vi "trial code.vi"() -> ()   [LabVIEW 2025]
uses:
  <vilib>/Instr/_visa.llb/VISA Configure Serial Port (Instr).vi
  <vilib>/addons/control/pid/NI_PID_pid.lvlib
  <vilib>/addons/control/pid/pid.llb/PID (DBL).vi
  <vilib>/numeric/Random Number (Range) DBL.vi
panel:
  in  "lower bound (0)":dbl
  in  "Stroke 2":dbl
  out "error out":errorcluster
  out "Stroke RAW":dbl
  out "Stroke Tare":dbl
  in  "Boolean":bool
  in  "PID SEND":bool
  in  "PID ON":bool
  in  "Stop 3":bool
  out "output Vpp":dbl
  in  "input variable":dbl=1.0
  in  "Stop 2":bool
  out "Stroke":dbl
  out "cof":dbl
  out "Friction":dbl
  out "pizo raw":dbl
  out "LVDT Peak":dbl
  out "LVDT MAX":dbl
  out "LVDT MIN":dbl
  in  "Stroke PID Gains 2":T1={"Proportional Gain (Kc)"=200.0, "Integral Time (Ti, min)"=0.02, "Derivative Time (Td, min)"=0.0}
  in  "STROKE GAIN :":dbl=700.0 caption="Stroke Gain :"
  in  "Set Strk":dbl=1.0 caption="STROKE LENGTH" min=1.0 max=1.0 step=1.0 format="%.3f"
  in  "PID Rst":bool=TRUE
  out "Stroke PID OUT":dbl(slide)=-13.483146067415703 scale=-600.0..600.0
  out "stop cmd":bool
  out "st gain":string="0000"
  out "PID Out":u8(slide) scale=0.0..4095.0
  out "start en":bool=TRUE
  in  "command":string
  in  "Stop":bool
  in  "Com Port 2":refnum<visa-resource-name>="COM9" caption="C2 :"
  out "Residual Uno 2":string
  out "Port 1 Error 2":errorcluster={"status"=TRUE, "code"=-1073807343, "source"="Property Node (arg 1) in VISA Configure Serial Port (Instr).vi->Winducom 2010--std ed hfrr-wo1768-V18.vi"}
  out "Uno Stroke":string
  out "Sps 4":dbl
  out "Port 1a 2":bool caption="Port 1 a"
  out "Port 2":u32(graph)
  out "Error Uno 2":errorcluster={"status"=TRUE, "code"=-1073807343, "source"="Property Node (arg 1) in VISA Configure Serial Port (Instr).vi->Winducom 2010--std ed hfrr-wo1768-V18.vi"}
  out "Port 4":bool=TRUE caption="Port 1"
  in  "Re-initialize Port1 2":bool
  out "Residual Uno":string
  out "Port 1 Error":errorcluster={"status"=TRUE, "code"=-1073807343, "source"="Property Node (arg 1) in VISA Configure Serial Port (Instr).vi->Winducom 2010--std ed hfrr-wo1768-V18.vi"}
  out "due":string
  out "Sps 3":dbl
  out "Port 1a":bool caption="Port 1 a"
  out "Port 1":u32(graph)
  out "Error Uno":errorcluster={"status"=TRUE, "code"=-1073807343, "source"="Property Node (arg 1) in VISA Configure Serial Port (Instr).vi->Winducom 2010--std ed hfrr-wo1768-V18.vi"}
  out "Port 3":bool=TRUE caption="Port 1"
  in  "Re-initialize Port1":bool
  out "FF buffer":dbl[](graph)
  in  "Com Port 1":refnum<visa-resource-name>="COM7" caption="C1 :"
  out "Test \nStatus":bool caption="Test Status"
types:
  T1 = cluster{"Proportional Gain (Kc)":dbl, "Integral Time (Ti, min)":dbl, "Derivative Time (Td, min)":dbl}
  T2 = cluster{"Read Heave and Surge":string, "Bytes at Heave Port":dbl, "Heave and Surge COM Port:":refnum<visa-resource-name>, "Com Port 2":refnum<visa-resource-name>, "Residual Due":string, "Heave COM Status 2":bool, "Heave COM Status":bool, "Port 2":bool, "Sway PPR":dbl, "Surge PPR":dbl, "Heave PPR":dbl, "Sway Pitch":dbl, "Surge Pitch":dbl, "Heave Pitch":dbl, "Sway Pulses/mm":dbl, "Surge Pulses/mm":dbl, "Heave Pulses/mm":dbl, "inner loop":dbl, "Read Heave and Surge 2":string, "String 36":string, "Write S":bool, "WriteCC1":string[], "Heave COM Loop":i32, "LastCom":string, "EXIT":bool, "Error Heave":errorcluster}
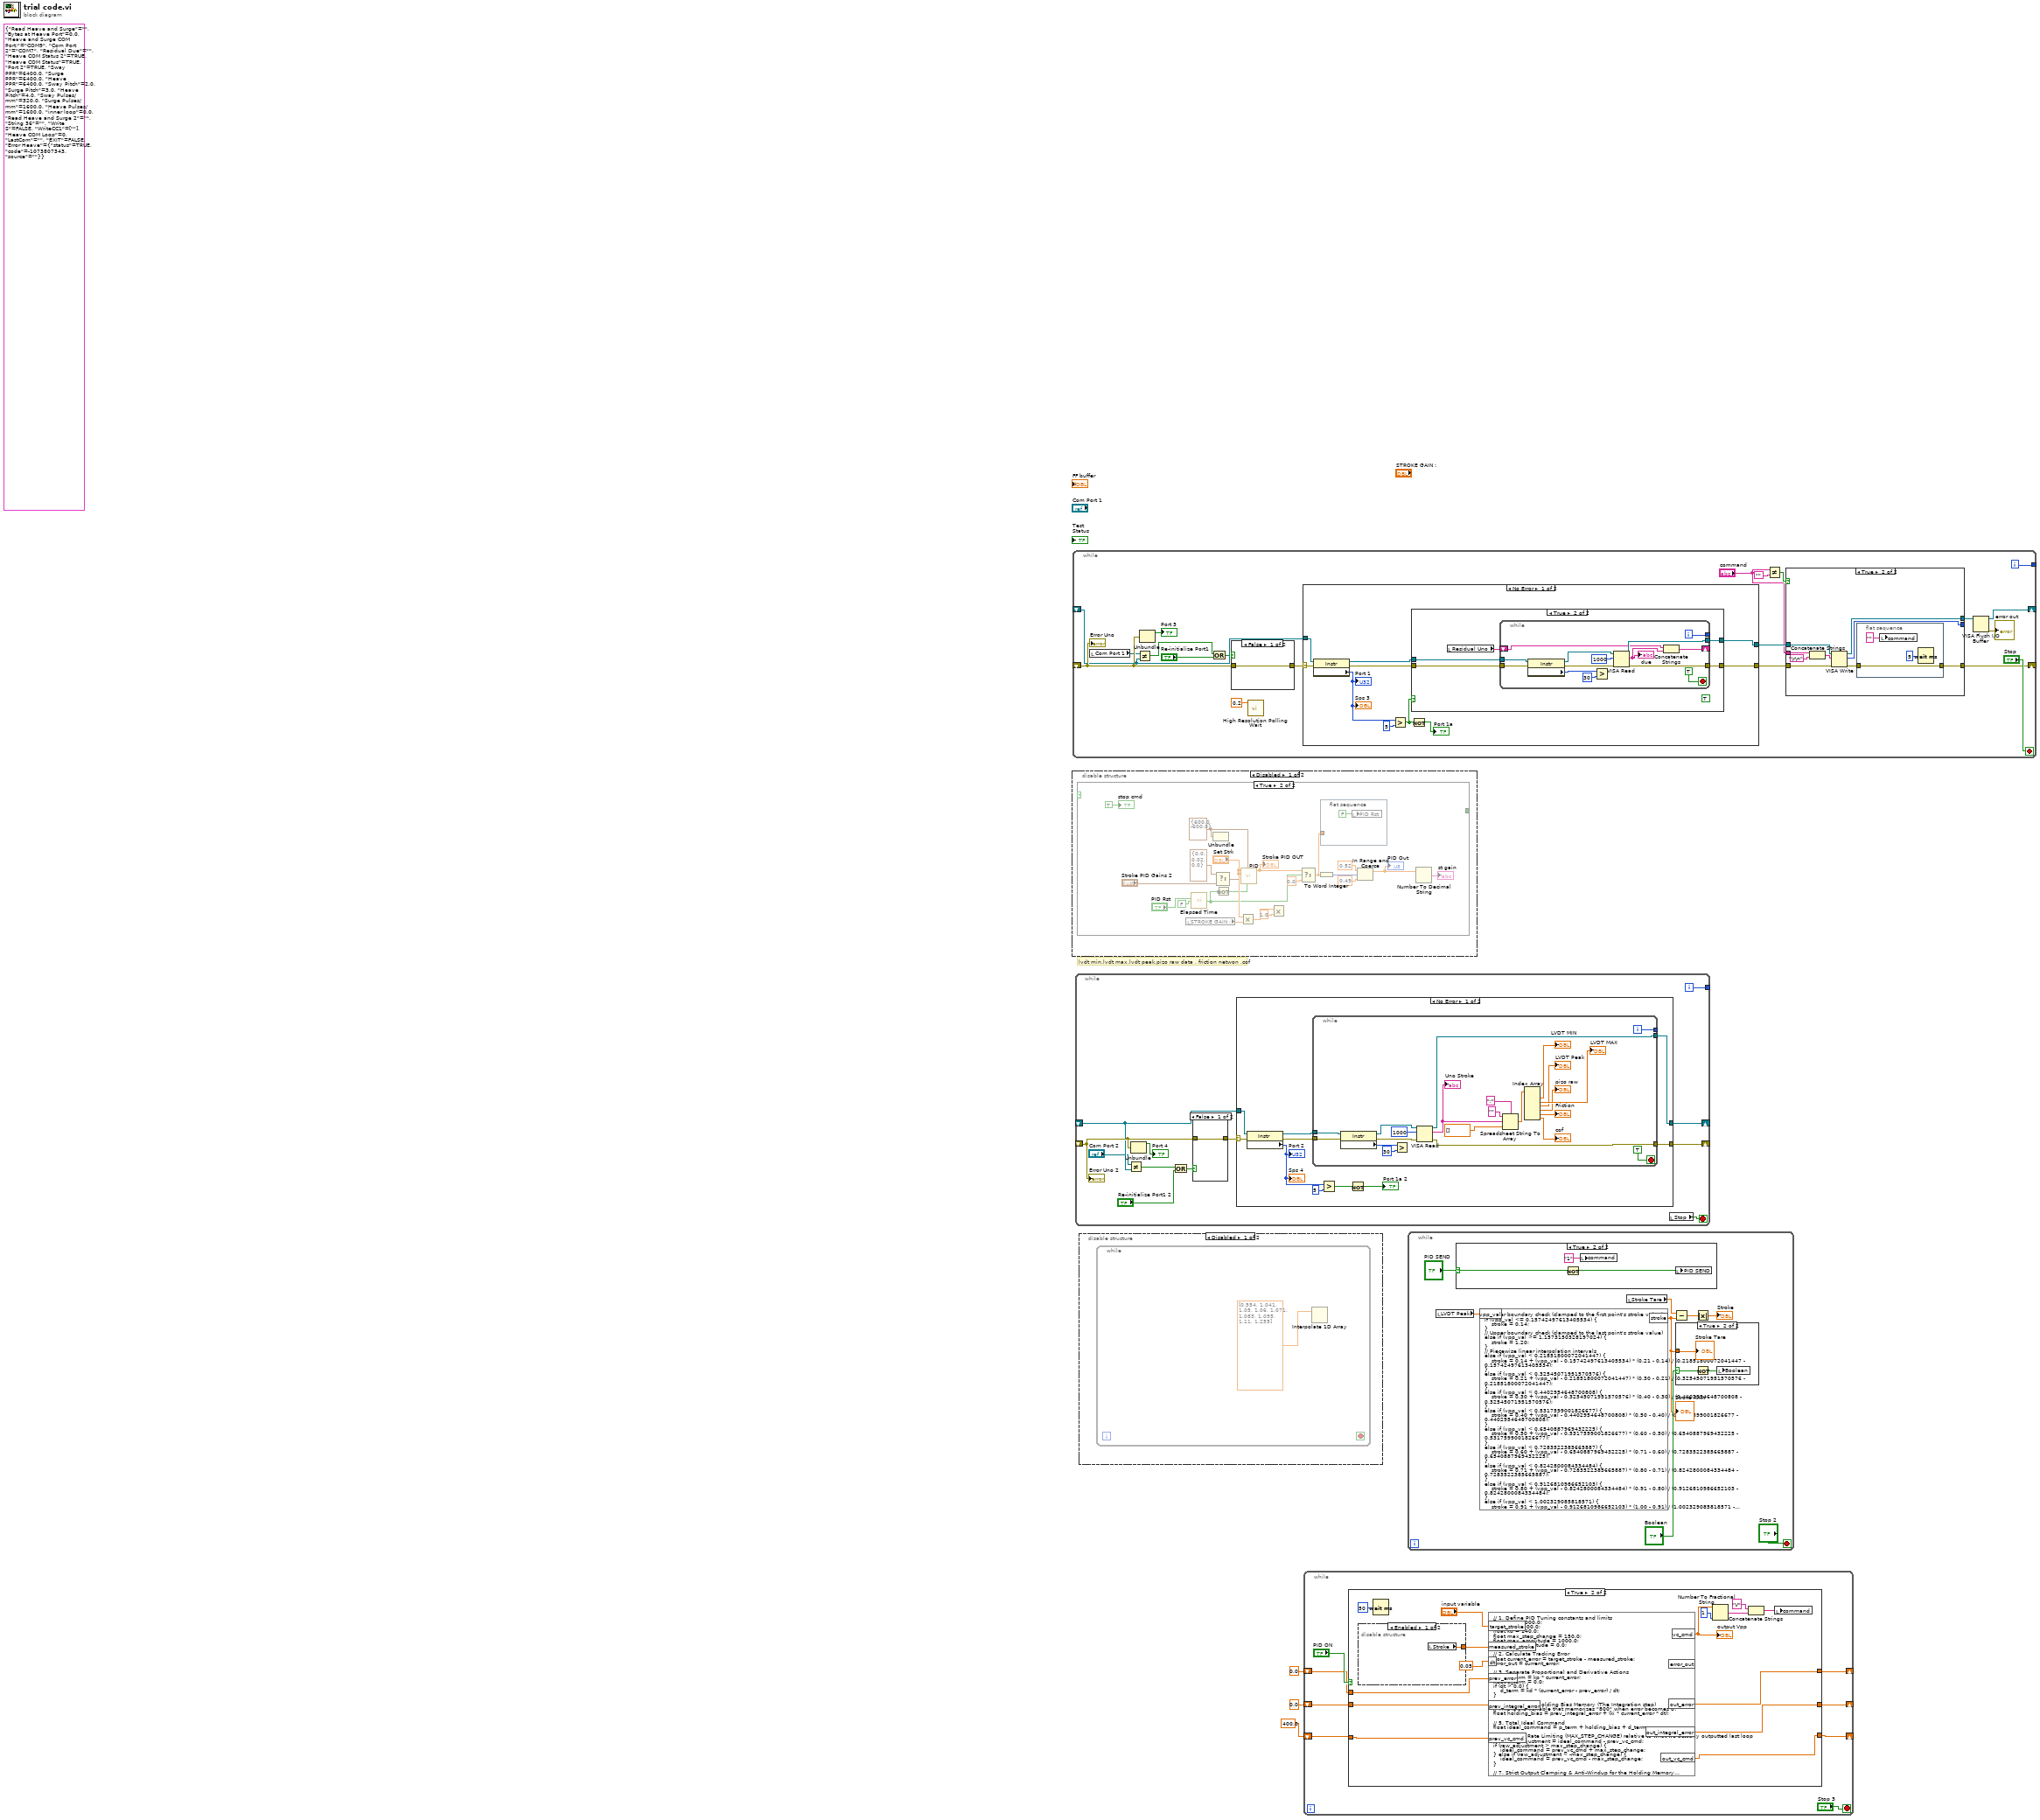
[diagram p0: block diagram]
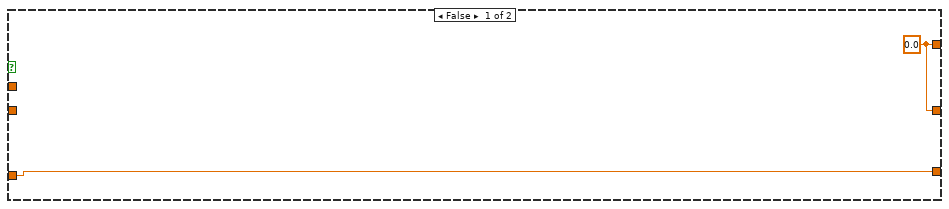
[diagram p2: hidden frame]
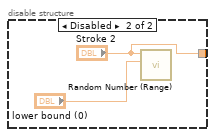
[diagram p3: hidden frame]
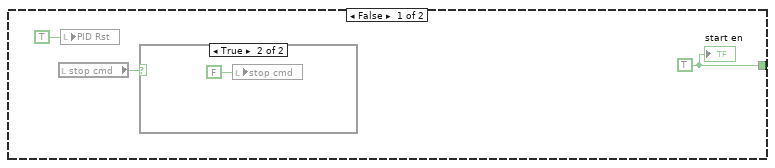
[diagram p7: hidden frame]
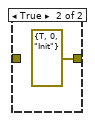
[diagram p10: hidden frame]
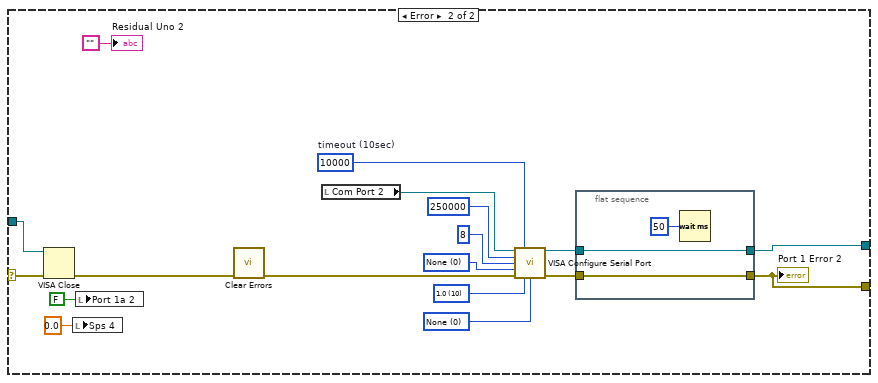
[diagram p11: hidden frame]
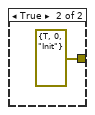
[diagram p13: hidden frame]
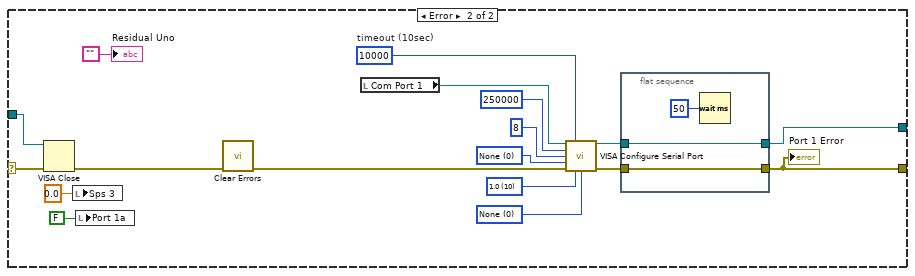
[diagram p15: hidden frame]
diagram:
  (unwired) T2 {"Read Heave and Surge"="", "Bytes at Heave Port"=0.0, "Heave and Surge COM Port:"="COM9", "Com Port 2"="COM7", "Residual Due"="", "Heave COM Status 2"=TRUE, "Heave COM Status"=TRUE, "Port 2"=TRUE, "Sway PPR"=6400.0, "Surge PPR"=6400.0, "Heave PPR"=6400.0, "Sway Pitch"=2.0, "Surge Pitch"=3.0, "Heave Pitch"=4.0, "Sway Pulses/mm"=320.0, "Surge Pulses/mm"=1600.0, "Heave Pulses/mm"=1600.0, "inner loop"=0.0, "Read Heave and Surge 2"="", "String 36"="", "Write S"=FALSE, "WriteCC1"=[""], "Heave COM Loop"=0, "LastCom"="", "EXIT"=FALSE, "Error Heave"={"status"=TRUE, "code"=-1073807343, "source"=""}}
  # "lvdt min,lvdt max,lvdt peak,pizo raw data , friction netwon ,cof"
  n1 = disable-structure shown="Disabled" {
    frame Disabled {
      n2 = case shown="True" {
        selector: _ -> [_ _]
        tunnel: [w4 _] -> _
        frame False {
          w4 = TRUE ("PID Rst")
          n3 = local read "stop cmd"() -> (w5:bool)
          n4 = local write "PID Rst"(TRUE ("PID Rst")) -> ()
          n5 = case shown="True" w5 {
            frame False {
            }
            frame True {
              n6 = local write "stop cmd"(FALSE ("stop cmd")) -> ()
            }
          }
          "start en" <- w4
        }
        frame True {
          w24 = cluster{"output high":dbl, "output low":dbl} {"output high"=600.0, "output low"=-600.0} ("output range")
          n7 = local read "STROKE GAIN :"() -> (w14:dbl)
          n8 = call "Elapsed Time"("Reset"="PID Rst", "Auto Reset"=FALSE) -> ("Time has Elapsed"=w21:bool)  [unwired: 10 in, 7 out]
          n9 = Unbundle(w24) -> ()  [unwired: 2 out]
          n10 = Select(t=T1 {"Proportional Gain (Kc)"=0.0, "Integral Time (Ti, min)"=0.02, "Derivative Time (Td, min)"=0.0} ("Stroke PID Gains"), f="Stroke PID Gains 2") -> (s? t:f=w11:T1)  [unwired: 1 in]
          n11 = Not(x=w21) -> (.not. x?=w20:bool)
          n12 = Multiply(x="Set Strk", y=w14) -> (x*y=w9:dbl)
          n13 = call-poly <vilib>:"PID.vi"("reinitialize? (F)"=w20, "output range"=w24, "PID gains"=w11, "process variable"="Set Strk", "setpoint"="Set Strk") -> ("output"=w19:dbl)  [unwired: 5 in, 1 out]
          "Stroke PID OUT" <- w19
          n14 = Multiply(x=w9, y=1.0) -> ()  [unwired: 1 out]
          n15 = Select(t=w19, s=w21, f=0.0) -> (s? t:f=w22:dbl)
          n16 = To Word Integer(number=w22) -> (16bit integer=w16:i16)
          n17 = flat-sequence {
            tunnel: w22 -> [_]
            frame #0 {
              n18 = local write "PID Rst"(FALSE ("PID Rst")) -> ()
            }
          }
          n19 = In Range and Coerce(upper limit=0.52 ("f"), x=w16, lower limit=0.49 ("f")) -> (coerced(x)=w13:dbl)  [unwired: 1 out]
          "PID Out" <- w13
          n20 = Number To Decimal String(number=w13) -> (decimal integer string=→"st gain":string)  [unwired: 1 in]
          "stop cmd" <- TRUE ("Auto Reset")
        }
      }
    }
    frame Enabled {
    }
  }
  n21 = while {
    shift-right: [w31] -> _
    shift-left: _ -> [w45]
    shift-right: [w36] -> _
    shift-left: _ -> [w47]
    tunnel: [w49] -> _
    i -> [w49]
    stop <- "Stop" stop-if-true
    n22 = local read "Com Port 1"() -> (w46:refnum<visa-resource-name>)
    n23 = Not Equal?(x=w46, y=w45) -> (x != y?=w44:bool)
    n24 = Unbundle(w47) -> ("status"=→"Port 3":bool)  [unwired: 2 out]
    n25 = Or(x=w44, y="Re-initialize Port1") -> (x .or. y?=w42:bool)
    n26 = case shown="False" w42 {
      tunnel: [w64 errorcluster {"status"=TRUE, "code"=0, "source"="Init"} ("error out")] -> w43
      tunnel: w47 -> [w64 _]
      frame False {
      }
      frame True {
      }
    }
    n27 = call <vilib>:"High Resolution Polling Wait.vi"("seconds to wait"=0.2) -> ()  [unwired: 10 in, 1 out]
    n28 = case shown="No Error" w43 {
      selector: w43 -> [w72 w102]
      tunnel: [w75 w106] -> w37
      tunnel: [w74 w99] -> w38
      tunnel: w45 -> [w73 w104]
      frame No Error {
        n29 = property class="Instr"(reference=w73, error in=w72) -> (reference out=w70:refnum<visa-resource-name>, error out=w71:errorcluster, "Serial Settings:Number of Bytes at Serial Port"=w66:u32)
        "Sps 3" <- w66
        "Port 1" <- w66
        n30 = Greater?(x=w66, y=u32 5) -> (0:w68:bool)
        n31 = Not(x=w68) -> (.not. x?=→"Port 1a":bool)
        n32 = case shown="True" w68 {
          tunnel: w70 -> [w77 w81]
          tunnel: w71 -> [w76 w79]
          tunnel: [w76 w78] -> w74
          tunnel: [w77 w82] -> w75
          frame False {
          }
          frame True {
            (unwired) TRUE ("PAUSE")
            n33 = local read "Residual Uno"() -> (w80:string)
            n34 = while {
              tunnel: [w94] -> w78
              tunnel: [w93] -> w82
              tunnel: w79 -> [w92]
              tunnel: w81 -> [w91]
              tunnel: [w89] -> _
              shift-right: [w86] -> _
              shift-left: w80 -> [w87]
              i -> [w89]
              stop <- TRUE stop-if-true
              n35 = property class="Instr"(reference=w91, error in=w92) -> (reference out=w96:refnum<visa-resource-name>, error out=w95:errorcluster, "Serial Settings:Number of Bytes at Serial Port"=w88:u32)
              n36 = Greater?(x=w88, y=u32 30) -> ()  [unwired: 1 out]
              n37 = VISA Read(VISA resource name=w96, byte count=u32 1000, error in (no error)=w95) -> (VISA resource name out=w93:refnum<visa-resource-name>, read buffer=w83:string, error out=w94:errorcluster)  [unwired: 1 out]
              "due" <- w83
              n38 = Concatenate Strings(w87, w83) -> (w86:string)
            }
          }
        }
      }
      frame Error {
        w112 = u16 0 items=["None", "XON/XOFF", "RTS/CTS", "XON/XOFF & RTS/CTS", "DTR/DSR", "XON/XOFF & DTR/DSR"] ("flow control (0:none)  2")
        w110 = u16 10 items=["1.0"=10, "1.5"=15, "2.0"=20] ("stop bits 2")
        w108 = u16 0 items=["None", "Odd", "Even", "Mark", "Space"] ("parity 2")
        w109 = u32 10000  # timeout (10sec)
        n39 = VISA Close(VISA resource name=w104, error in (no error)=w102) -> (error out=w105:errorcluster)
        n40 = local write "Sps 3"(0.0 ("Sps 4")) -> ()
        n41 = local write "Port 1a"(FALSE ("Port 1a")) -> ()
        n42 = call <vilib>:"Clear Errors.vi"("error in (no error)"=w105) -> ("error out"=w103:errorcluster)  [unwired: 5 in, 1 out]
        n43 = local read "Com Port 1"() -> (w98:refnum<visa-resource-name>)
        n44 = call-poly "VISA Configure Serial Port"("VISA resource name"=w98, "timeout (10sec)"=w109, "baud rate (9600)"=u32 250000 ("baud rate  2"), "data bits (8)"=u16 8 ("data bits  2"), "parity (0:none)"=w108, "error in (no error)"=w103, "stop bits (10: 1 bit)"=w110, "flow control (0:none)"=w112) -> ("VISA resource name out"=w113:refnum<visa-resource-name>, "error out"=w114:errorcluster)  [unwired: 6 in]
        n45 = flat-sequence {
          tunnel: w113 -> [w116]
          tunnel: w114 -> [w115]
          tunnel: [w116] -> w106
          tunnel: [w115] -> w99
          frame #0 {
            n46 = Wait (ms)(milliseconds to wait=u32 50) -> ()  [unwired: 1 out]
          }
        }
        "Residual Uno" <- ""
        "Port 1 Error" <- w99
      }
    }
    n47 = Not Equal?(x="command", y="") -> (x != y?=w33:bool)
    n48 = case shown="True" w33 {
      tunnel: w37 -> [w51 w56]
      tunnel: [w51 w60] -> w35
      tunnel: w38 -> [w50 w55]
      tunnel: [w50 w58] -> w36
      tunnel: "command" -> [_ w54]
      tunnel: [_ w57] -> _
      frame False {
        # "DATA  WRITE LOOP"
      }
      frame True {
        n49 = Concatenate Strings(w54, "\r\n") -> (w53:string)
        n50 = VISA Write(VISA resource name=w56, write buffer=w53, error in (no error)=w55) -> (VISA resource name out=w60:refnum<visa-resource-name>, return count=w57:u32, error out=w59:errorcluster)
        n51 = flat-sequence {
          tunnel: w59 -> [w62]
          tunnel: [w62] -> w58
          frame #0 {
            n52 = local write "command"("" ("command")) -> ()
            n53 = Wait (ms)(milliseconds to wait=u32 5) -> ()  [unwired: 1 out]
          }
        }
      }
    }
    n54 = VISA Flush I/O Buffer(VISA resource name=w35) -> (VISA resource name out=w31:refnum<visa-resource-name>, error out=→"error out":errorcluster)  [unwired: 2 in]
    "Error Uno" <- w47
  }
  n55 = while {
    shift-right: [w129] -> _
    shift-left: _ -> [w124]
    shift-right: [w128] -> _
    shift-left: _ -> [w125]
    tunnel: [w127] -> _
    i -> [w127]
    stop <- w118 stop-if-true
    n56 = Not Equal?(x="Com Port 2", y=w124) -> (x != y?=w123:bool)
    n57 = Unbundle(w125) -> ("status"=→"Port 4":bool)  [unwired: 2 out]
    n58 = Or(x=w123, y="Re-initialize Port1 2") -> (x .or. y?=w121:bool)
    n59 = case shown="False" w121 {
      tunnel: [w130 errorcluster {"status"=TRUE, "code"=0, "source"="Init"} ("error out")] -> w122
      tunnel: w125 -> [w130 _]
      frame False {
      }
      frame True {
      }
    }
    n60 = case shown="No Error" w122 {
      selector: w122 -> [w138 w169]
      tunnel: [w141 w173] -> w129
      tunnel: [w140 w166] -> w128
      tunnel: w124 -> [w139 w171]
      frame No Error {
        n61 = property class="Instr"(reference=w139, error in=w138) -> (reference out=w136:refnum<visa-resource-name>, error out=w137:errorcluster, "Serial Settings:Number of Bytes at Serial Port"=w132:u32)
        "Sps 4" <- w132
        "Port 2" <- w132
        n62 = while {
          tunnel: [w161] -> w140
          tunnel: [w160] -> w141
          tunnel: w137 -> [w159]
          tunnel: w136 -> [w158]
          tunnel: [w156] -> _
          i -> [w156]
          stop <- TRUE stop-if-true
          n63 = property class="Instr"(reference=w158, error in=w159) -> (reference out=w163:refnum<visa-resource-name>, error out=w162:errorcluster, "Serial Settings:Number of Bytes at Serial Port"=w155:u32)
          n64 = Greater?(x=w155, y=u32 30) -> ()  [unwired: 1 out]
          n65 = VISA Read(VISA resource name=w163, byte count=u32 1000, error in (no error)=w162) -> (VISA resource name out=w160:refnum<visa-resource-name>, read buffer=w152:string, error out=w161:errorcluster)  [unwired: 1 out]
          "Uno Stroke" <- w152
          n66 = Spreadsheet String To Array(delimiter (Tab)=";", format string="", spreadsheet string=w152, array type (2D Dbl)=dbl[] []) -> (array=w149:dbl[])
          n67 = Index Array(array=w149) -> (element #1=→"LVDT MIN":dbl, element #2=→"LVDT MAX":dbl, element #3=→"LVDT Peak":dbl, element #4=→"pizo raw":dbl, element #5=→"Friction":dbl, element #6=→"cof":dbl)  [unwired: 6 in]
        }
        n68 = Greater?(x=w132, y=u32 5) -> (0:w134:bool)
        n69 = Not(x=w134) -> (.not. x?=→"Port 1a 2":bool)
      }
      frame Error {
        w179 = u16 0 items=["None", "XON/XOFF", "RTS/CTS", "XON/XOFF & RTS/CTS", "DTR/DSR", "XON/XOFF & DTR/DSR"] ("flow control (0:none)  2")
        w177 = u16 10 items=["1.0"=10, "1.5"=15, "2.0"=20] ("stop bits 2")
        w175 = u16 0 items=["None", "Odd", "Even", "Mark", "Space"] ("parity 2")
        w176 = u32 10000  # timeout (10sec)
        n70 = VISA Close(VISA resource name=w171, error in (no error)=w169) -> (error out=w172:errorcluster)
        n71 = local write "Sps 4"(0.0 ("Sps 4")) -> ()
        n72 = local write "Port 1a 2"(FALSE ("Port 1a")) -> ()
        n73 = call <vilib>:"Clear Errors.vi"("error in (no error)"=w172) -> ("error out"=w170:errorcluster)  [unwired: 5 in, 1 out]
        n74 = local read "Com Port 2"() -> (w164:refnum<visa-resource-name>)
        n75 = call-poly "VISA Configure Serial Port"("VISA resource name"=w164, "timeout (10sec)"=w176, "baud rate (9600)"=u32 250000 ("baud rate  2"), "data bits (8)"=u16 8 ("data bits  2"), "parity (0:none)"=w175, "error in (no error)"=w170, "stop bits (10: 1 bit)"=w177, "flow control (0:none)"=w179) -> ("VISA resource name out"=w180:refnum<visa-resource-name>, "error out"=w181:errorcluster)  [unwired: 6 in]
        n76 = flat-sequence {
          tunnel: w180 -> [w183]
          tunnel: w181 -> [w182]
          tunnel: [w183] -> w173
          tunnel: [w182] -> w166
          frame #0 {
            n77 = Wait (ms)(milliseconds to wait=u32 50) -> ()  [unwired: 1 out]
          }
        }
        "Residual Uno 2" <- ""
        "Port 1 Error 2" <- w166
      }
    }
    n78 = local read "Stop"() -> (w118:bool)
    "Error Uno 2" <- w125
  }
  n79 = disable-structure shown="Disabled" {
    frame Disabled {
      n80 = while {
        stop <- _ stop-if-true
        n81 = Interpolate 1D Array(2:dbl[] [0.554, 1.041, 1.05, 1.06, 1.071, 1.083, 1.095, 1.11, 1.255] ("array of numbers or points")) -> ()  [unwired: 1 in, 1 out]
      }
    }
    frame Enabled {
    }
  }
  n82 = while {
    shift-right: [w187] -> _
    shift-left: 0.0 -> [w190]
    shift-right: [w186] -> _
    shift-left: 0.0 -> [w189]
    shift-right: [w188] -> _
    shift-left: 400.0 ("vc_cmd") -> [w193]
    stop <- "Stop 3" stop-if-true
    n83 = case shown="True" "PID ON" {
      tunnel: w193 -> [w195 w201]
      tunnel: w190 -> [_ w199]
      tunnel: w189 -> [_ w200]
      tunnel: [w195 w198] -> w188
      tunnel: [w194 w197] -> w187
      tunnel: [w194 w196] -> w186
      frame False {
        w194 = 0.0 ("error_out")
      }
      frame True {
        n84 = disable-structure shown="Enabled" {
          disable-tunnel: [w211 "Stroke 2"] -> w209
          frame Enabled {
            n85 = local read "Stroke"() -> (w211:dbl)
          }
          frame Disabled {
            n86 = call-poly <vilib>:"Random Number (Range).vi"("lower bound (0)"="lower bound (0)", "upper bound (100)"="Stroke 2") -> ()  [unwired: 9 in, 1 out]
          }
        }
        n87 = Wait (ms)(milliseconds to wait=u32 50) -> ()  [unwired: 1 out]
        n88 = formula code="// 1. Define PID Tuning constants and limits\nfloat kp = 2000.0;\nfloat ki = 1300.0;\nfloat kd = 140.0;\nfloat max_step_change = 150.0;\nfloat max_amplitude = 1000.0; \nfloat min_amplitude = 0.0;\n\n// 2. Calculate Tracking Error\nfloat current_error = target_stroke - measured_stroke;\nerror_out = current_error; \n\n// 3. Separate Proportional and Derivative Actions\nfloat p_term = kp * current_error;\nfloat d_term = 0.0;\nif (dt > 0.0) {\n    d_term = kd * (current_error - prev_error) / dt;\n}\n\n// 4. Update the Holding Bias Memory (The Integration step)\n// This is the variable that memorizes \"800\" when error becomes 0!\nfloat holding_bias = prev_integral_error + (ki * current_error * dt);\n\n// 5. Total Ideal Command\nfloat ideal_command = p_term + holding_bias + d_term;\n\n// 6. Enforce Rate Limiting (MAX_STEP_CHANGE) relative to what we actually outputted last loop\nfloat raw_adjustment = ideal_command - prev_vc_cmd;\nif (raw_adjustment > max_step_change) {\n    ideal_command = prev_vc_cmd + max_step_change;\n} else if (raw_adjustment < -max_step_change) {\n    ideal_command = prev_vc_cmd - max_step_change;\n}\n\n// 7. Strict Output Clamping & Anti-Windup for the Holding Memory\nvc_cmd = ideal_command;\nif (vc_cmd > max_amplitude) {\n    vc_cmd = max_amplitude;\n    holding_bias = prev_integral_error; // Freeze memory if saturated\n} else if (vc_cmd < min_amplitude) {\n    vc_cmd = min_amplitude;\n    holding_bias = prev_integral_error; // Freeze memory if saturated\n}\n\n// 8. Map to Shift Registers for the next iteration\nout_error = current_error;\nout_integral_error = holding_bias; // Save the memorized voltage step\nout_vc_cmd = vc_cmd;"("target_stroke"="input variable", "measured_stroke"=w209, "dt"=0.05 ("input variable"), "prev_integral_error"=w199, "prev_error"=w200, "prev_vc_cmd"=w201) -> ("vc_cmd"=w206:dbl, "out_error"=w196:dbl, "out_integral_error"=w197:dbl, "out_vc_cmd"=w198:dbl)  [unwired: 1 out]
        "output Vpp" <- w206
        n89 = Number To Fractional String(number=w206, precision (6)=i16 1) -> (F-format string=w204:string)  [unwired: 2 in]
        n90 = Concatenate Strings("V" ("string"), w204) -> (w202:string)
        n91 = local write "command"(w202) -> ()
      }
    }
  }
  n92 = while {
    stop <- "Stop 2" stop-if-true
    n93 = local read "LVDT Peak"() -> (w221:dbl)
    n94 = case shown="True" "PID SEND" {
      selector: "PID SEND" -> [_ w227]
      frame False {
      }
      frame True {
        n95 = Not(x=w227) -> (.not. x?=w226:bool)
        n96 = local write "command"("1" ("command")) -> ()
        n97 = local write "PID SEND"(w226) -> ()
      }
    }
    n98 = formula code="// Lower boundary check (clamped to the first point's stroke value)\nif (vpp_val <= 0.15742497613405534) {\n    stroke = 0.14;\n} \n// Upper boundary check (clamped to the last point's stroke value)\nelse if (vpp_val >= 1.1573150328197024) {\n    stroke = 1.20;\n} \n// Piecewise linear interpolation intervals\nelse if (vpp_val < 0.21851800072041447) {\n    stroke = 0.14 + (vpp_val - 0.15742497613405534) * (0.21 - 0.14) / (0.21851800072041447 - 0.15742497613405534);\n} \nelse if (vpp_val < 0.32545071951570576) {\n    stroke = 0.21 + (vpp_val - 0.21851800072041447) * (0.30 - 0.21) / (0.32545071951570576 - 0.21851800072041447);\n} \nelse if (vpp_val < 0.4402954648700808) {\n    stroke = 0.30 + (vpp_val - 0.32545071951570576) * (0.40 - 0.30) / (0.4402954648700808 - 0.32545071951570576);\n} \nelse if (vpp_val < 0.5317599001826677) {\n    stroke = 0.40 + (vpp_val - 0.4402954648700808) * (0.50 - 0.40) / (0.5317599001826677 - 0.4402954648700808);\n} \nelse if (vpp_val < 0.6540887969432225) {\n    stroke = 0.50 + (vpp_val - 0.5317599001826677) * (0.60 - 0.50) / (0.6540887969432225 - 0.5317599001826677);\n} \nelse if (vpp_val < 0.7283522385665887) {\n    stroke = 0.60 + (vpp_val - 0.6540887969432225) * (0.71 - 0.60) / (0.7283522385665887 - 0.6540887969432225);\n} \nelse if (vpp_val < 0.8242800084334484) {\n    stroke = 0.71 + (vpp_val - 0.7283522385665887) * (0.80 - 0.71) / (0.8242800084334484 - 0.7283522385665887);\n} \nelse if (vpp_val < 0.9126810986652103) {\n    stroke = 0.80 + (vpp_val - 0.8242800084334484) * (0.91 - 0.80) / (0.9126810986652103 - 0.8242800084334484);\n} \nelse if (vpp_val < 1.002329085818571) {\n    stroke = 0.91 + (vpp_val - 0.9126810986652103) * (1.00 - 0.91) / (1.002329085818571 - 0.9126810986652103);\n} \nelse if (vpp_val < 1.0872106603548073) {\n    stroke = 1.00 + (vpp_val - 1.002329085818571) * (1.11 - 1.00) / (1.0872106603548073 - 1.002329085818571);\n} \nelse {\n    // This final block covers: 1.0872106603548073 <= vpp_val < 1.1573150328197024\n    stroke = 1.11 + (vpp_val - 1.0872106603548073) * (1.20 - 1.11) / (1.1573150328197024 - 1.0872106603548073);\n}"("vpp_val"=w221) -> ("stroke"=w216:dbl)
    "Stroke RAW" <- w216
    n99 = local read "Stroke Tare"() -> (w217:dbl)
    n100 = Subtract(x=w217, y=w216) -> (x-y=w215:dbl)
    n101 = case shown="True" "Boolean" {
      selector: "Boolean" -> [_ w224]
      tunnel: w216 -> [_ w222]
      frame False {
      }
      frame True {
        n102 = Not(x=w224) -> (.not. x?=w223:bool)
        n103 = local write "Boolean"(w223) -> ()
        "Stroke Tare" <- w222
      }
    }
    n104 = Absolute Value(x=w215) -> (abs(x)=→"Stroke":dbl)
  }
